vi "UpdateHealthAndStatus.vi"(0 "InternalHealthAndStatusFIFO":refnum<k21>="txModbusPort1FIFO", 5 "AddressOffset":u32, 7 "BaseAddress":u32, 9 "HealthAndStatusUpdateMode":T1, 11 "Data":u64) -> ()   [LabVIEW 2018, in "FPGAHealthAndStatus.lvlib"]
uses:
  FPGAHealthAndStatus.lvlib
  DataTypes/HealthAndStatusUpdateMode.ctl
  DataTypes/HealthAndStatusUpdate.ctl
  <vilib>/rvi/DataTransferAndStorage/Container/Common/niFpgaContainerExecOnDevCompGetState.vi
  <vilib>/rvi/Emulation/niFpgaEmulationIsFPGAContextNoSignature.vi
  <vilib>/rvi/Emulation/niFpgaSctlEmulationGetInTimedLoop.vi
  <vilib>/rvi/errors/niFpgaSetErrorForExecOnDevCompSimple.vi
  <vilib>/rvi/eio/common/nirviEmuReportErrorAndStop.vi
  <vilib>/rvi/DataTransferAndStorage/Container/Common/niFpgaContainerGetUniqueNameForEmu.vi
  <vilib>/rvi/FIFO/Fifo_Resource/nirvififoEmulationSetSize.vi
  <vilib>/rvi/FIFO/Fifo_Resource/nirviFifoEmulationQueueMgr.vi
  <instcachedir>/0/nirviFifoEmulationQueueMgr_E5CAEC123FF24DC58D834DCA3CDAA9B5.lvgen/nirviFifoEmulationQueueMgr_E5CAEC123FF24DC58D834DCA3CDAA9B5_018.vi
  <vilib>/rvi/FIFO/Fifo_Resource/nirvififoEmulationDetermineInputValidOut.vi
  <vilib>/rvi/FIFO/Fifo_Resource/nirvififoEmulationCreateLock.vi
  <vilib>/rvi/Emulation/niFpgaProcessEmulError.vi
  <vilib>/rvi/FIFO/Fifo_Resource/nirvififoEmulationObtainLock.vi
  <vilib>/rvi/FIFO/Fifo_Resource/nirvififoEmulationReleaseLock.vi
  <vilib>/rvi/occurrence/nirviWaitOnOccurrenceBase.vi
  <vilib>/rvi/errors/nirviReportUnexpectedCaseInternalError.vi
  <vilib>/rvi/errors/nirviReportUnexpectedCaseInternalError (U32).vi
  <vilib>/Utility/error.llb/Clear Errors.vi
  <vilib>/rvi/interface/RandomDataEmulation/niFpgaRandomDataHandleErrors.vi
  <vilib>/rvi/DataTransferAndStorage/Container/XNode/niFpgaContainer.xnode
  <vilib>/rvi/FIFO/Fifo_Resource/niFpgaFifoEmulationRefIn.vi
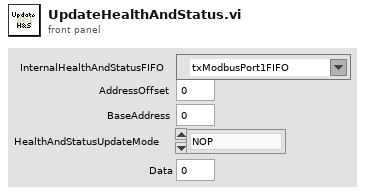
[diagram p1: front panel]
types:
  T1 = typedef "FPGAHealthAndStatus.lvlib/HealthAndStatusUpdateMode.ctl" = enum8{"NOP", "Set", "Add", "Subtract", "Or", "Not And"}
  T2 = typedef "FPGAHealthAndStatus.lvlib/HealthAndStatusUpdate.ctl" = cluster{"Address":u32, "UpdateMode":T1, "Data":u64}
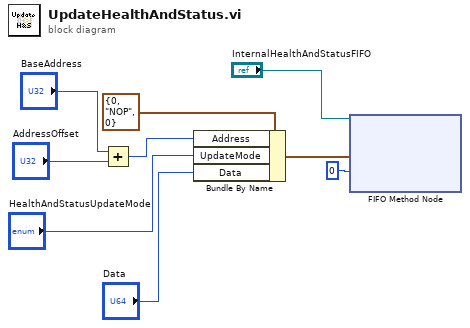
[diagram p0: block diagram]
diagram:
  n1 = Add(x="BaseAddress", y="AddressOffset") -> (x+y=w4:u32)
  n2 = Bundle By Name(cluster=T2 {"Address"=0, "UpdateMode"=enum."NOP", "Data"=0} ("Telemetry Update"), "Address"=w4, "UpdateMode"="HealthAndStatusUpdateMode", "Data"="Data") -> (w2:T2)
  n3 = xnode ("FIFO Method Node")("Element"=w2, "Timeout"=0, "FIFO In"="InternalHealthAndStatusFIFO") -> ()  [unwired: 2 out]
